vi "Cleanup.vi"(8 "error in {ignored}":errorcluster, 11 "Object Dictionary":refnum<class "objdict.lvclass">) -> (0 "error out":errorcluster)   [LabVIEW 2015, in "objdict.lvclass"]
doc: "Cleans up the object dictionary by destroying all Data Value References holding its member objects.\n\n<b>This VI is unsafe:</b> The member objects are not returned by this VI, so you can't call their cleanup methods if they have them. If the member objects need to be cleaned up, remove each one from the dictionary meanually. The <b>Clean Up Dictionary Objects.vit</b> template is available on the palette to make that easier."
uses:
  objdict.lvclass
  objdict.lvclass/objdict.ctl
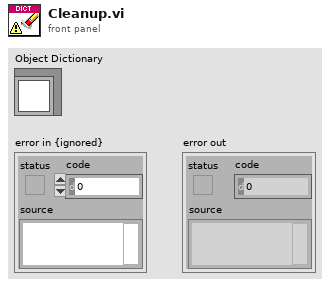
[diagram p1: front panel]
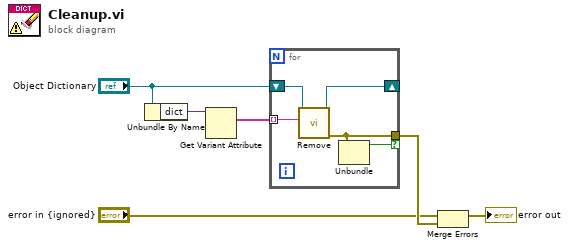
[diagram p0: block diagram]
diagram:
  n1 = Unbundle By Name("Object Dictionary") -> ("dict"=w6:variant)
  n2 = Get Variant Attribute(Variant=w6) -> (names=w4:string[])  [unwired: 3 in, 3 out]
  n3 = for {
    tunnel: w4 -> [w11] mode=indexing
    shift-right: [w9] -> _
    shift-left: "Object Dictionary" -> [w10]
    tunnel: [w8] -> w5 if=w7
    n4 = call "Remove.vi"("key"=w11, "Object Dictionary in"=w10) -> ("error out"=w8:errorcluster, "Object Dictionary out"=w9:refnum<class "objdict.lvclass">)  [unwired: 6 in, 2 out]
    n5 = Unbundle(w8) -> ("status"=w7:bool)  [unwired: 2 out]
  }
  n6 = Merge Errors("error in {ignored}", w5) -> (→"error out":errorcluster)
